vi "Open.vi"(6 "timeout":i32=20, 8 "error in (no error)":errorcluster, 10 "nbaud":i32=9600, 11 "Serial Port":string) -> (0 "error out":errorcluster, 3 "hDevice":i32, 5 "Connected?":bool)   [LabVIEW 2018, in "Thorlabs_SC10.lvlib"]
doc: "Open com port."
uses:
  Thorlabs_SC10.lvlib
  SC10CommandLib_x64.dll
  SC10CommandLib_win32.dll
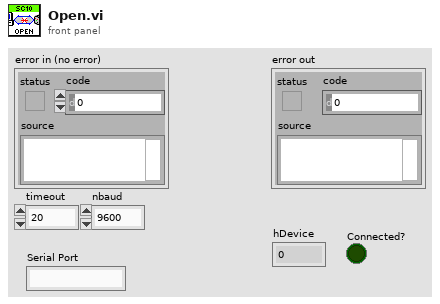
[diagram p1: front panel]
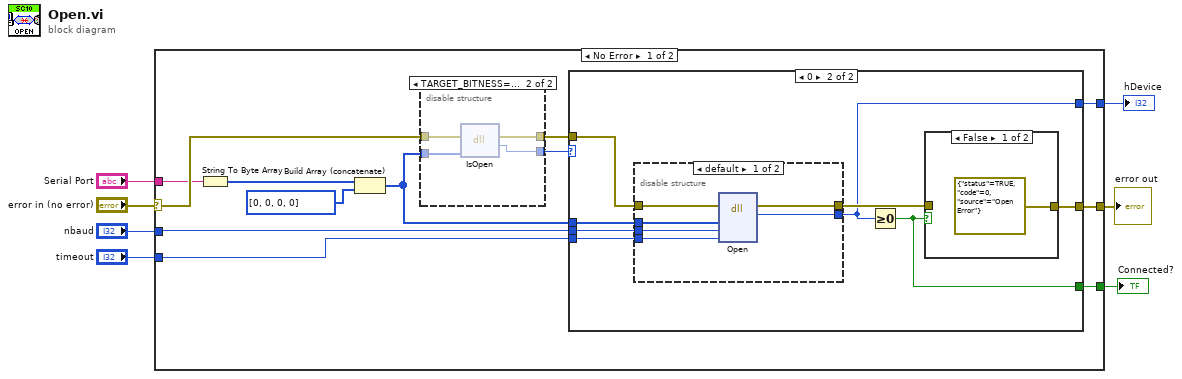
[diagram p0: block diagram]
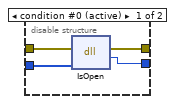
[diagram p2: hidden frame]
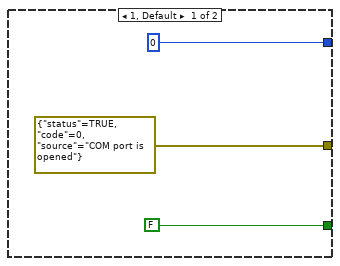
[diagram p3: hidden frame]
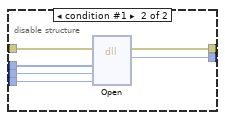
[diagram p4: hidden frame]
diagram:
  n1 = case shown="No Error" "error in (no error)" {
    selector: "error in (no error)" -> [w14 w53]
    tunnel: [w19 w53] -> w6
    tunnel: "timeout" -> [w17 _]
    tunnel: "nbaud" -> [w18 _]
    tunnel: "Serial Port" -> [w11 _]
    tunnel: [w16 _] -> w2
    tunnel: [w15 _] -> w1
    frame No Error {
      n2 = String To Byte Array(string=w11) -> (unsigned byte array=w10:u8[])
      n3 = Build Array (concatenate)(w10, u8[] [0, 0, 0, 0] ("array")) -> (w9:u8[])
      n4 = disable-structure shown="TARGET_BITNESS==64" {
        disable-tunnel: w9 -> [w23 w27]
        disable-tunnel: w14 -> [w22 w26]
        disable-tunnel: [w21 w25] -> w13
        disable-tunnel: [w20 w24] -> w12
        frame condition #0 (active) {
          n5 = dll-call lib="C:/Program Files (x86)/National Instruments/LabVIEW 2018/instr.lib/Thorlabs_SC10/Data/SC10CommandLib_win32.dll" fn="IsOpen"(error in=w22, "Serial Number"=w23) -> (error out=w21:errorcluster, "return type"=w20:i32)  [unwired: 3 in, 1 out]
        }
        frame condition #1 {
          n6 = dll-call lib="C:/Program Files/National Instruments/LabVIEW 2011/instr.lib/Thorlabs_SC10/Data/SC10CommandLib_x64.dll" fn="IsOpen"(error in=w26, "Serial Number"=w27) -> (error out=w25:errorcluster, "return type"=w24:i32)  [unwired: 3 in, 1 out]
        }
      }
      n7 = case shown="0" w12 {
        tunnel: [errorcluster {"status"=TRUE, "code"=0, "source"="COM port is opened"} ("error out") w38] -> w19
        tunnel: w18 -> [_ w37]
        tunnel: w17 -> [_ w36]
        tunnel: [0 ("return type") w34] -> w16
        tunnel: [FALSE w33] -> w15
        tunnel: w9 -> [_ w32]
        tunnel: w13 -> [_ w31]
        frame 1, Default {
        }
        frame 0 {
          n8 = disable-structure shown="default" {
            disable-tunnel: w37 -> [w44 w50]
            disable-tunnel: w36 -> [w43 w49]
            disable-tunnel: [w42 w48] -> w35
            disable-tunnel: [w41 w47] -> w34
            disable-tunnel: w32 -> [w40 w46]
            disable-tunnel: w31 -> [w39 w45]
            frame condition #0 (active) {
              n9 = dll-call lib="C:/Program Files (x86)/National Instruments/LabVIEW 2018/instr.lib/Thorlabs_SC10/Data/SC10CommandLib_win32.dll" fn="Open"(error in=w39, "Serial Number"=w40, "nbaud"=w44, "timeout"=w43) -> (error out=w42:errorcluster, "return type"=w41:i32)  [unwired: 5 in, 1 out]
            }
            frame condition #1 {
              n10 = dll-call lib="C:/Program Files/National Instruments/LabVIEW 2011/instr.lib/Thorlabs_SC10/Data/SC10CommandLib_x64.dll" fn="Open"(error in=w45, "Serial Number"=w46, "nbaud"=w50, "timeout"=w49) -> (error out=w48:errorcluster, "return type"=w47:i32)  [unwired: 5 in, 1 out]
            }
          }
          n11 = Greater Or Equal To 0?(x=w34) -> (x >= 0?=w33:bool)
          n12 = case shown="False" w33 {
            tunnel: w35 -> [_ w52]
            tunnel: [errorcluster {"status"=TRUE, "code"=0, "source"="Open Error"} ("error out") w52] -> w38
            frame False {
            }
            frame True {
            }
          }
        }
      }
    }
    frame Error {
    }
  }
  "error out" <- w6
  "hDevice" <- w2
  "Connected?" <- w1
